vi "Ready_measurement.vi"(10 "discharge time (ms)":u32=250, 11 "VISA resource name":refnum<visa-resource-name>="COM4") -> (3 "VISA resource name out":refnum<visa-resource-name>)   [LabVIEW 2024]
uses:
  support/Serial - XON-XOFF Characters.ctl
  support/Serial - ASCII Characters.ctl
  support/Serial - Settings.ctl
  <vilib>/Instr/_visa.llb/VISA Configure Serial Port (Instr).vi
panel:
  # "• When the path pointer detects a colon (:), it moves down to the next command level. An exception is when the path pointer detects a semicolon (;), which is used to separate commands within the program message. \n• When the path pointer detects a colon (:) that immediately follows a semicolon (;), it resets to the root level. \n• The path pointer can only move down. It cannot be moved up a level. Executing a command at a higher level requires that you start over at the root command."
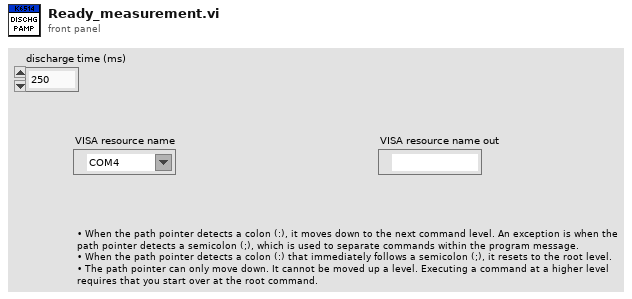
[diagram p1: front panel]
types:
  T1 = typedef "Serial - Settings.ctl" = cluster{"baud rate":u32, "data bits":u16, "parity":enum16{"None", "Odd", "Even", "Mark", "Space"}, "stop bits":u16, "flow control":u16}
  T2 = typedef "Serial - XON-XOFF Characters.ctl" = cluster{"XON":T3, "XOFF":T3}
  T3 = typedef "Serial - ASCII Characters.ctl" = enum16{"NUL", "SOH", "STX", "ETX", "EOT", "ENQ", "ACK", "BEL", "BS", "HT", "LF", "VT", "FF", "CR", "SO", "SI", "DLE", "DC1", "DC2", "DC3", "DC4", "NAK", "SYN", "ETB", "CAN", "EM", "SUB", "ESC", "FS", "GS", "RS", "US", "SP", "!", "\"", "#", "$", "%", "&", "'", "(", ")", "*", "+", ",", "- (-)", ".", "/", "0", "1", "2", "3", "4", "5", "6", "7", "8", "9", ":", ";", "<", "=", ">", "?", "@", "A", "B", "C", "D", "E", "F", "G", "H", "I", "J", "K", "L", "M", "N", "O", "P", "Q", "R", "S", "T", "U", "V", "W", "X", "Y", "Z", "[", "\\", "]", "^", "_", "`", "a", "b", "c", "d", "e", "f", "g", "h", "i", "j", "k", "l", "m", "n", "o", "p", "q", "r", "s", "t", "u", "v", "w", "x", "y", "z", "{", "|", "}", "~"}
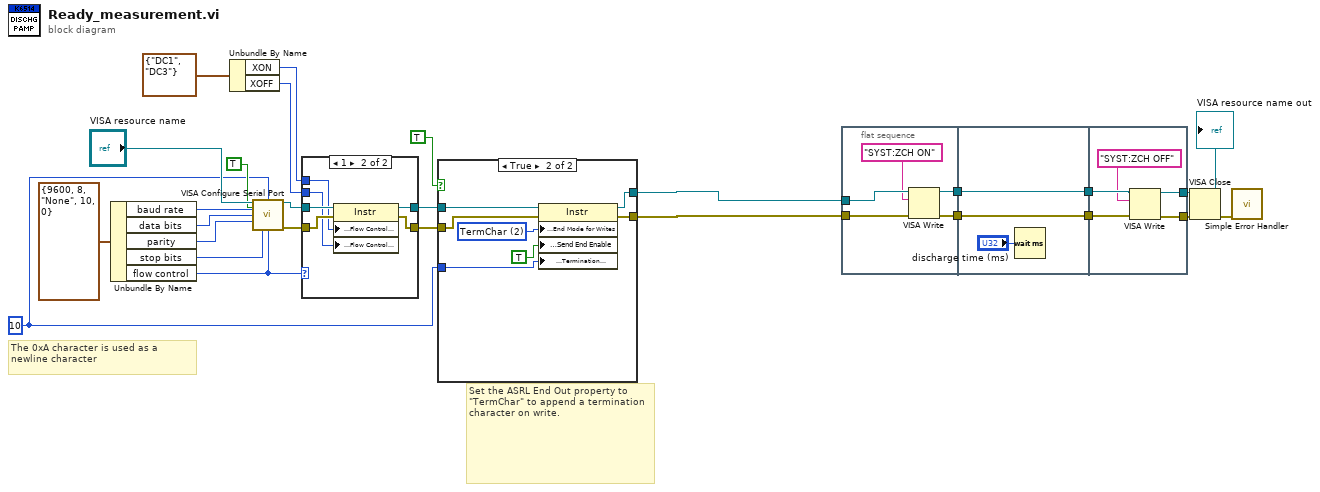
[diagram p0: block diagram]
diagram:
  w10 = u8 10 ("Termination Character")
  # "The 0xA character is used as a newline character"
  # "Set the ASRL End Out property to \"TermChar\" to append a termination character on write."
  n1 = Unbundle By Name(T1 {"baud rate"=9600, "data bits"=8, "parity"=enum."None", "stop bits"=10, "flow control"=0} ("Serial Settings")) -> ("baud rate"=w19:u32, "data bits"=w20:u16, "parity"=w21:enum16{"None", "Odd", "Even", "Mark", "Space"}, "stop bits"=w22:u16, "flow control"=w16:u16)
  n2 = Unbundle By Name(T2 {"XON"=enum."DC1", "XOFF"=enum."DC3"} ("XON/XOFF Characters")) -> ("XON"=w15:T3, "XOFF"=w14:T3)
  n3 = call-poly "VISA Configure Serial Port"("VISA resource name"="VISA resource name", "termination char\n(0xA = '\\n' = LF)"=w10, "Enable Termination\nChar (T)"=TRUE ("End Read on Termination Character?"), "baud rate (9600)"=w19, "data bits (8)"=w20, "parity (0:none)"=w21, "stop bits (10: 1 bit)"=w22, "flow control (0:none)"=w16) -> ("VISA resource name out"=w23:refnum<visa-resource-name>, "error out"=w24:errorcluster)  [unwired: 2 in, 4 out]
  n4 = case shown="1" w16 {
    tunnel: [w27 w34] -> w13
    tunnel: [w28 w33] -> w12
    tunnel: w24 -> [w27 w32]
    tunnel: w23 -> [w28 w31]
    tunnel: w15 -> [_ w30]
    tunnel: w14 -> [_ w29]
    frame Default {
    }
    frame 1 {
      n5 = property class="Instr"(reference=w31, error in=w32, "Serial Settings:Flow Control XON Character"=w30, "Serial Settings:Flow Control XOFF Character"=w29) -> (reference out=w33:refnum<visa-resource-name>, error out=w34:errorcluster)
    }
  }
  n6 = case shown="True" TRUE ("End Write on Termination Character?") {
    tunnel: w12 -> [w35 w43]
    tunnel: w13 -> [w36 w42]
    tunnel: [w35 w41] -> w8
    tunnel: [w36 w40] -> w7
    tunnel: w10 -> [_ w38]
    frame False {
    }
    frame True {
      w39 = u16 2 items=["None", "LastBit", "TermChar", "Break"] ("Serial Settings:Serial End Mode for Writes")
      n7 = property class="Instr"(reference=w43, error in=w42, "Serial Settings:End Mode for Writes"=w39, "Message Based Settings:Send End Enable"=TRUE, "Message Based Settings:Termination Character"=w38) -> (reference out=w41:refnum<visa-resource-name>, error out=w40:errorcluster)
    }
  }
  n8 = flat-sequence {
    tunnel: w8 -> [w48]
    tunnel: w7 -> [w47]
    tunnel: [w46] -> w5
    tunnel: [w45] -> w3
    tunnel: [w51] -> w6
    tunnel: w5 -> [w51]
    tunnel: [w50] -> w4
    tunnel: w3 -> [w50]
    tunnel: w6 -> [w56]
    tunnel: w4 -> [w55]
    tunnel: [w53] -> w2
    tunnel: [w52] -> w1
    frame #0 {
      n9 = VISA Write(VISA resource name=w48, write buffer="SYST:ZCH ON" ("String"), error in (no error)=w47) -> (VISA resource name out=w46:refnum<visa-resource-name>, error out=w45:errorcluster)  [unwired: 1 out]
    }
    frame #1 {
      n10 = Wait (ms)(milliseconds to wait="discharge time (ms)") -> ()  [unwired: 1 out]
    }
    frame #2 {
      n11 = VISA Write(VISA resource name=w56, write buffer="SYST:ZCH OFF", error in (no error)=w55) -> (VISA resource name out=w53:refnum<visa-resource-name>, error out=w52:errorcluster)  [unwired: 1 out]
    }
  }
  n12 = VISA Close(VISA resource name=w2, error in (no error)=w1) -> (error out=w9:errorcluster)
  n13 = call <vilib>:"Simple Error Handler.vi"("error in (no error)"=w9) -> ()  [unwired: 1 in, 8 out]
  "VISA resource name out" <- w2
